vi "Get Package BuildSpec (By Name).vi"(8 "error in (no error)":errorcluster, 10 "package build spec name":string, 11 "LabVIEW project filepath":path) -> (0 "error out":errorcluster, 2 "package build spec ref out":refnum<vi>, 3 "project ref out":refnum<vi>)   [LabVIEW 2018, in "NIPKG BuildSpec API.lvlib"]
uses:
  NIPKG BuildSpec API.lvlib
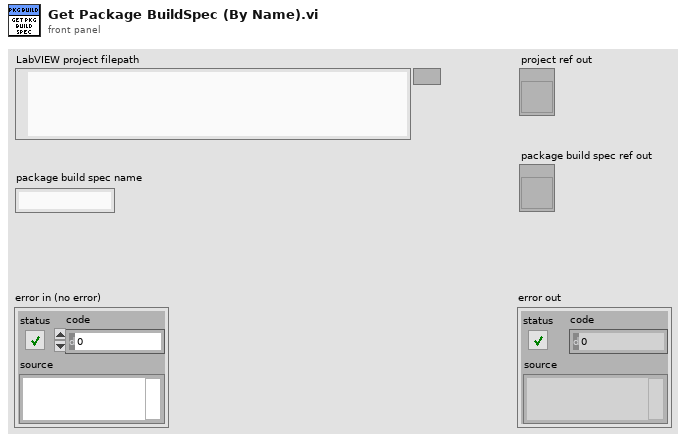
[diagram p1: front panel]
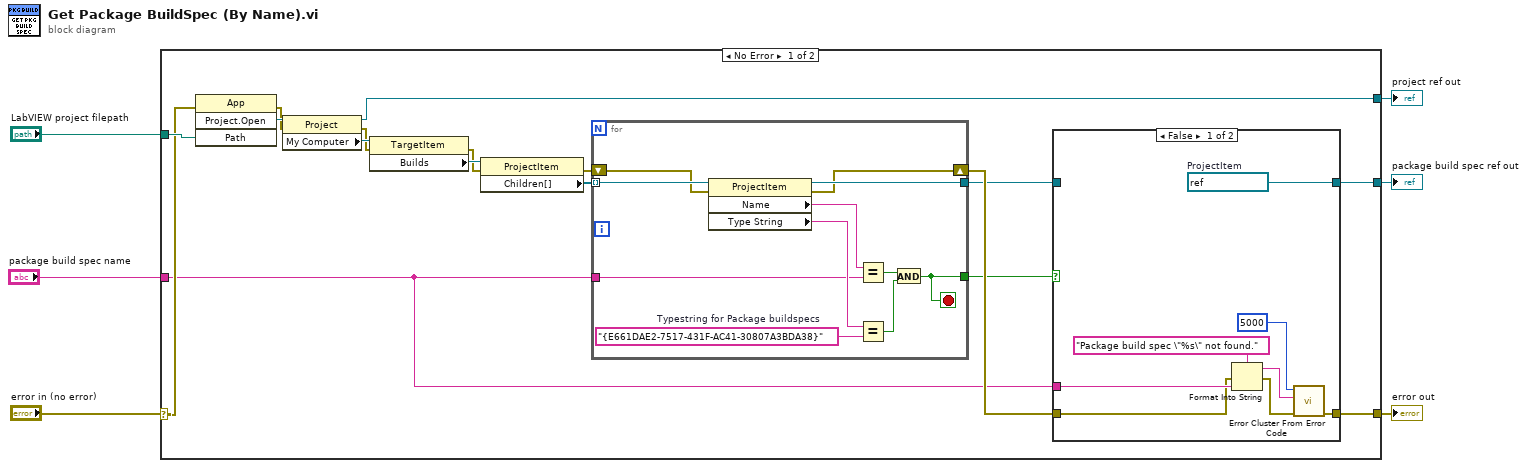
[diagram p0: block diagram]
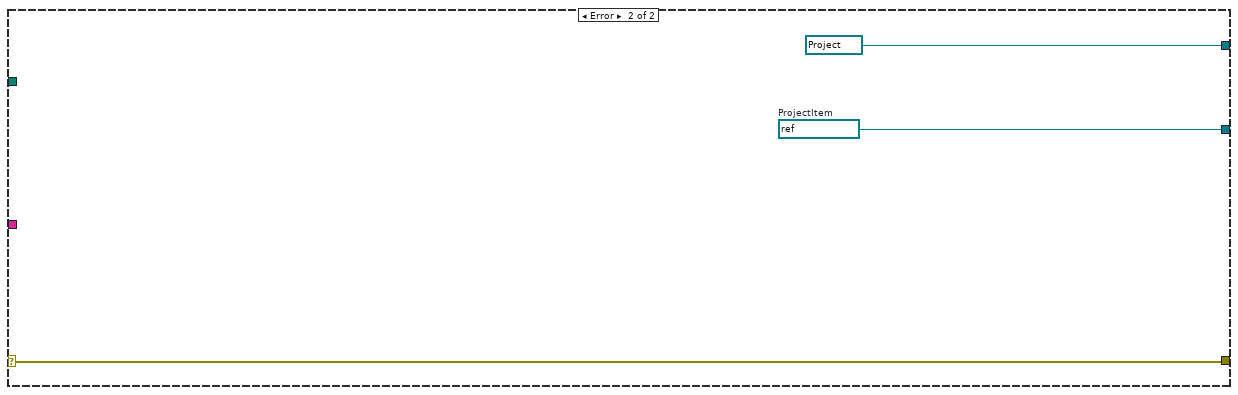
[diagram p3: hidden frame]
diagram:
  n1 = case shown="No Error" "error in (no error)" {
    selector: "error in (no error)" -> [w18 w47]
    tunnel: "LabVIEW project filepath" -> [w19 _]
    tunnel: [w11 w47] -> w4
    tunnel: [w12 refnum<vi> refnum ("Project:Open")] -> w3
    tunnel: [w7 w45] -> w2
    tunnel: "package build spec name" -> [w10 _]
    frame No Error {
      n2 = invoke class="App" method="Project.Open"(error in=w18, "Path"=w19) -> (error out=w17:errorcluster, "Project:Open"=w23:refnum<vi>)  [unwired: 2 in, 2 out]
      n3 = property class="Project"(reference=w23, error in=w17) -> (reference out=w12:refnum<vi>, error out=w16:errorcluster, "My Computer"=w22:refnum<vi>)
      n4 = property class="TargetItem"(reference=w22, error in=w16) -> (error out=w15:errorcluster, "Builds"=w21:refnum<vi>)  [unwired: 1 out]
      n5 = property class="ProjectItem"(reference=w21, error in=w15) -> (error out=w14:errorcluster, "Children[]"=w20:refnum<vi>[])  [unwired: 1 out]
      n6 = for {
        tunnel: w20 -> [w44] mode=indexing
        tunnel: [w41] -> w8
        shift-right: [w39] -> w13
        shift-left: w14 -> [w40]
        tunnel: w10 -> [w37]
        tunnel: [w34] -> w9
        stop <- w34 stop-if-true
        w42 = "{E661DAE2-7517-431F-AC41-30807A3BDA38}"  # Typestring for Package buildspecs
        n7 = property class="ProjectItem"(reference=w44, error in=w40) -> (reference out=w41:refnum<vi>, error out=w39:errorcluster, "Name"=w38:string, "Type String"=w43:string)
        n8 = Equal?(x=w38, y=w37) -> (x = y?=w36:bool)
        n9 = Equal?(x=w43, y=w42) -> (x = y?=w35:bool)
        n10 = And(x=w36, y=w35) -> (x .and. y?=w34:bool)
      }
      n11 = case shown="False" w9 {
        tunnel: w13 -> [w28 w33]
        tunnel: [w31 w33] -> w11
        tunnel: w10 -> [w29 _]
        tunnel: w8 -> [_ w32]
        tunnel: [w24 w32] -> w7
        frame False {
          w24 = refnum<vi> refnum  # ProjectItem
          n12 = Format Into String(format string="Package build spec \"%s\" not found.", error in=w28, w29) -> (resulting string=w26:string, error out=w27:errorcluster)  [unwired: 1 in]
          n13 = call <vilib>:"Error Cluster From Error Code.vi"("error in (no error)"=w27, "error message (\"\")"=w26, "error code (0)"=5000) -> ("error out"=w31:errorcluster)  [unwired: 6 in]
        }
        frame True {
        }
      }
    }
    frame Error {
      w45 = refnum<vi> refnum  # ProjectItem
    }
  }
  "error out" <- w4
  "project ref out" <- w3
  "package build spec ref out" <- w2
